vi "decode_incoming_data.vi"(9 "N":dbl, 10 "Input Data":u8[](array[numeric])=[63, 21]) -> (1 "Combined output binary values":u8[](array[numeric]) format="%b")   [LabVIEW 2012]
panel:
  out "array 0 size":dbl
  out "Output Araay Size":dbl
  out "Last incoming byte":u8
  out "Input Array Size":dbl
  out "Byte 2 array":u8[](array[numeric])
  out "Byte 1 array":u8[](array[numeric])
  out "Loop count":i32
  out "Byte 2":bool[](array[boolean])
  out "Byte 1":bool[](array[boolean])
  out "Byte 0":bool[](array[boolean])
  out "The last input byte":bool[](array[boolean])
  out "Loop Counter":dbl
  out "Byte 2":u8
  out "Byte 1":u8
  out "Byte 0":u8
  out "Byte 0 array":u8[](array[numeric])
  # "Each incoming byte has 3 bytes of data"
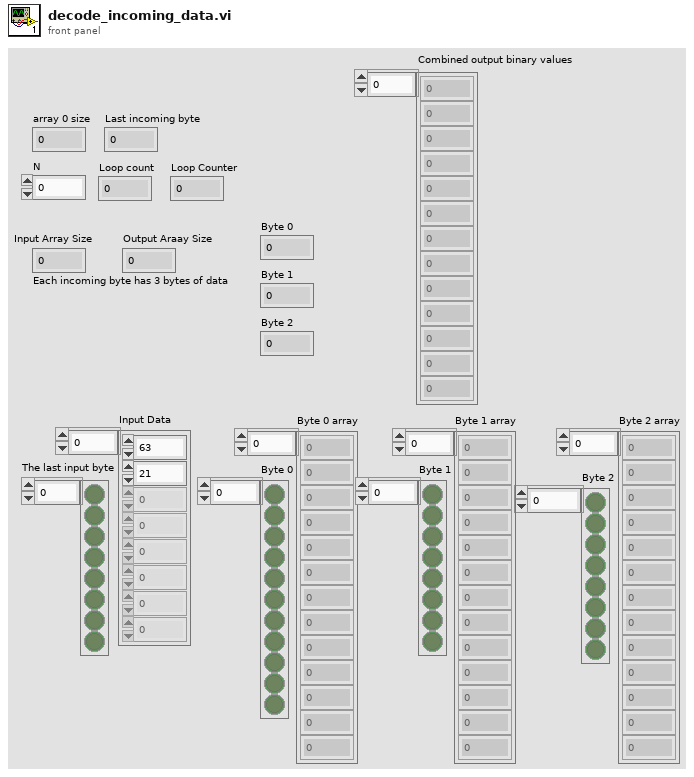
[diagram p1: front panel]
types:
  T1 = cluster{"Boolean array[0]":bool, "Boolean array[1]":bool, "Boolean array[2]":bool, "Boolean array[3]":bool, "Boolean array[4]":bool, "Boolean array[5]":bool, "Boolean array[6]":bool, "Boolean array[7]":bool}
  T2 = cluster{"Boolean array[0]":bool, "Boolean array[1]":bool, bool, bool, bool, bool, bool, bool}
  T3 = cluster{"Boolean array[2]":bool, "Boolean array[3]":bool, bool, bool, bool, bool, bool, bool}
  T4 = cluster{"Boolean array[4]":bool, "Boolean array[5]":bool, bool, bool, bool, bool, bool, bool}
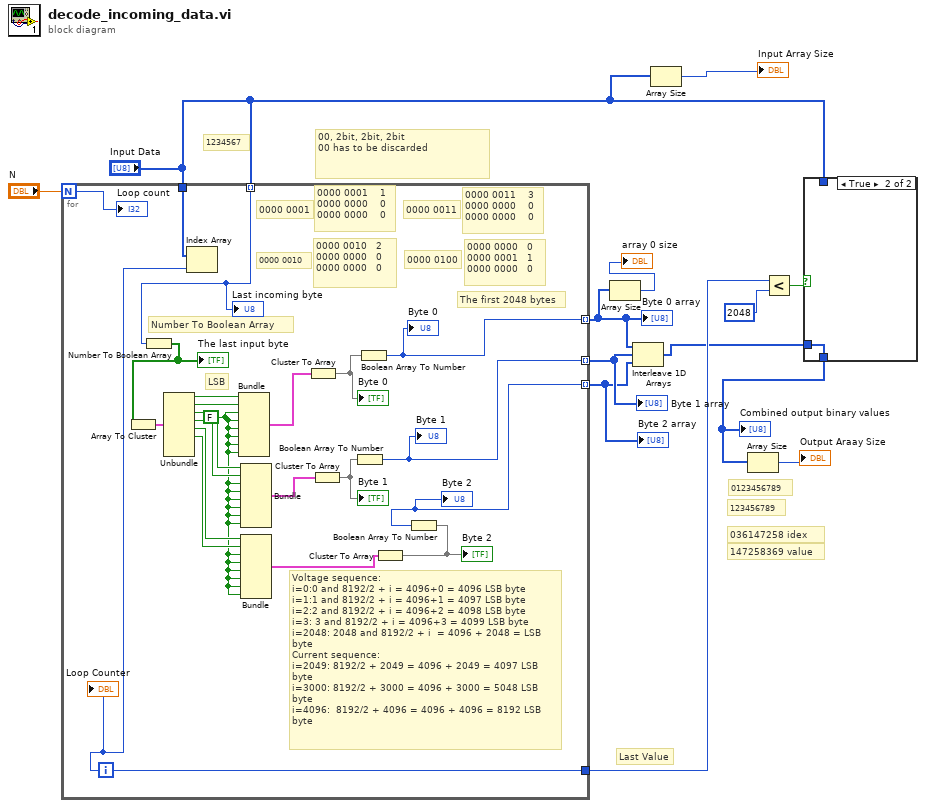
[diagram p0: block diagram]
diagram:
  # "1234567"
  # "036147258 idex"
  # "0123456789"
  # "147258369 value"
  # "123456789"
  # "00, 2bit, 2bit, 2bit\n00 has to be discarded"
  # "Last Value"
  n1 = for {
    N: "N" -> [w24]
    tunnel: "Input Data" -> [w23]
    tunnel: [w35] -> w3 mode=indexing
    tunnel: [w18] -> w11
    tunnel: "Input Data" -> [w19] mode=indexing
    tunnel: [w15] -> w2 mode=indexing
    tunnel: [w16] -> w4 mode=indexing
    i -> [w18]
    w20 = FALSE
    # "Number To Boolean Array"
    # "0000 0000   0\n0000 0001   1\n0000 0000   0"
    # "0000 0100"
    # "0000 0011    3\n0000 0000    0\n0000 0000    0"
    # "0000 0011"
    # "0000 0010   2\n0000 0000   0\n0000 0000   0"
    # "0000 0010"
    # "0000 0001    1\n0000 0000    0\n0000 0000    0"
    # "0000 0001"
    # "The first 2048 bytes"
    # "LSB"
    # "Voltage sequence:\ni=0:0 and 8192/2 + i = 4096+0 = 4096 LSB byte \ni=1:1 and 8192/2 + i = 4096+1 = 4097 LSB byte\ni=2:2 and 8192/2 + i = 4096+2 = 4098 LSB byte\ni=3: 3 and 8192/2 + i = 4096+3 = 4099 LSB byte\ni=2048: 2048 and 8192/2 + i  = 4096 + 2048 = LSB byte\nCurrent sequence:\ni=2049: 8192/2 + 2049 = 4096 + 2049 = 4097 LSB byte\ni=3000: 8192/2 + 3000 = 4096 + 3000 = 5048 LSB byte\ni=4096:  8192/2 + 4096 = 4096 + 4096 = 8192 LSB byte"
    n2 = Number To Boolean Array(number=w19) -> (Boolean array=w27:bool[])
    "The last input byte" <- w27
    n3 = Array To Cluster(array=w27) -> (cluster=w28:T1)
    n4 = Unbundle(w28) -> ("Boolean array[0]"=w34:bool, "Boolean array[1]"=w33:bool, "Boolean array[2]"=w32:bool, "Boolean array[3]"=w31:bool, "Boolean array[4]"=w30:bool, "Boolean array[5]"=w29:bool)  [unwired: 2 out]
    n5 = Index Array(array=w23, index=w18) -> ()  [unwired: 1 out]
    n6 = Bundle("Boolean array[0]"=w34, "Boolean array[1]"=w33, w20, w20, w20, w20, w20, w20) -> (w14:T2)  [unwired: 1 in]
    n7 = Bundle("Boolean array[2]"=w32, "Boolean array[3]"=w31, w20, w20, w20, w20, w20, w20) -> (w22:T3)  [unwired: 1 in]
    n8 = Bundle("Boolean array[4]"=w30, "Boolean array[5]"=w29, w20, w20, w20, w20, w20, w20) -> (w21:T4)  [unwired: 1 in]
    n9 = Cluster To Array(cluster=w14) -> (array=w17:bool[])
    "Byte 0" <- w17
    n10 = Cluster To Array(cluster=w22) -> (array=w26:bool[])
    "Byte 1" <- w26
    n11 = Boolean Array To Number(Boolean array=w26) -> (number=w16:u8)
    "Byte 1" <- w16
    n12 = Boolean Array To Number(Boolean array=w17) -> (number=w15:u8)
    "Byte 0" <- w15
    n13 = Cluster To Array(cluster=w21) -> (array=w25:bool[])
    "Byte 2" <- w25
    n14 = Boolean Array To Number(Boolean array=w25) -> (number=w35:u8)
    "Byte 2" <- w35
    "Loop Counter" <- w18
    "Loop count" <- w24
    "Last incoming byte" <- w19
  }
  "Byte 0 array" <- w2
  "Byte 1 array" <- w4
  "Byte 2 array" <- w3
  n15 = Array Size(array=w2) -> (size(s)=→"array 0 size":i32)
  n16 = Interleave 1D Arrays(w2, w4, w3) -> (w5:u8[])
  n17 = Array Size(array="Input Data") -> (size(s)=→"Input Array Size":i32)
  n18 = Less?(x=w11, y=2048) -> (x < y?=w12:bool)
  n19 = case shown="True" w12 {
    tunnel: "Input Data" -> [w36 _]
    tunnel: [w36 w37] -> w9
    tunnel: w5 -> [_ w37]
    frame False {
    }
    frame True {
    }
  }
  "Combined output binary values" <- w9
  n20 = Array Size(array=w9) -> (size(s)=→"Output Araay Size":i32)
